vi "Remote Start.vi"(8 "error in":errorcluster, 11 "Master Controller in":refnum<class "EMS User Interface.lvclass">) -> (0 "error out":errorcluster, 3 "Master Controller out":refnum<class "EMS User Interface.lvclass">)   [LabVIEW 2018, in "EMS User Interface Actor.lvlib" / "EMS User Interface.lvclass"]
uses:
  EMS User Interface.lvclass
  EMS User Interface.lvclass/EMS User Interface.ctl
  <vilib>/ActorFramework/Message Enqueuer/Message Enqueuer.lvclass/Message Enqueuer.ctl
  <vilib>/ActorFramework/Message Enqueuer/Enqueue.vi
  EMS Core/EMS Messages/Commissioning Init Msg/Commissioning Init Msg.lvclass
  C:/Program Files (x86)/National Instruments/LabVIEW 2018/vi.lib/ActorFramework/Message/Message.lvclass
  <vilib>/ActorFramework/Message Priority Queue/Priority Enqueue.vi
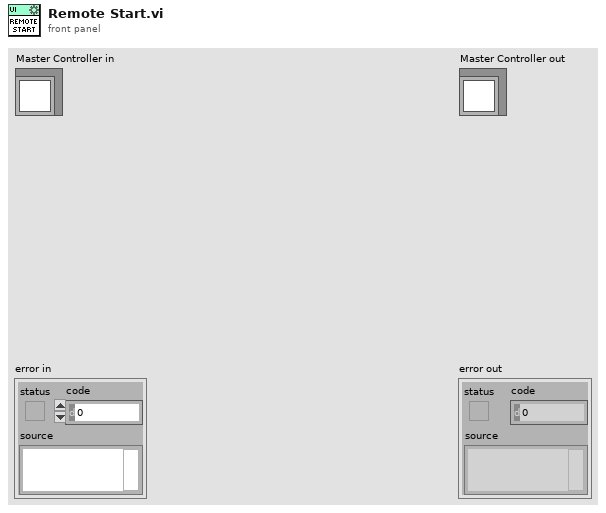
[diagram p1: front panel]
types:
  T1 = typedef "EMS Core.lvlib/EMS.lvclass/Microgrid State.ctl" = enum16{"Discovery", "Commissioning", "Activation", "Blackstart", "OnGrid", "OffGrid", "Island", "Resynchronization", "Manual", "Shutdown", "Stop"}
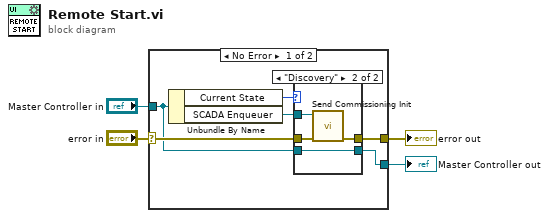
[diagram p0: block diagram]
diagram:
  n1 = case shown="No Error" "error in" {
    selector: "error in" -> [w9 w18]
    tunnel: [w10 w18] -> w2
    tunnel: [w8 w17] -> w1
    tunnel: "Master Controller in" -> [w6 w17]
    frame No Error {
      n2 = Unbundle By Name(w6) -> ("Current State"=w7:T1, "SCADA Enqueuer"=w5:refnum<class "Message Enqueuer.lvclass">)
      n3 = case shown="\"Discovery\"" w7 {
        tunnel: [w12 w14] -> w10
        tunnel: w6 -> [w11 w16]
        tunnel: w9 -> [w12 w15]
        tunnel: [w11 w16] -> w8
        tunnel: w5 -> [_ w13]
        frame "Shutdown", Default {
        }
        frame "Discovery" {
          n4 = call "Send Commissioning Init.vi"("error in (no error)"=w15, "Message Enqueuer"=w13) -> ("error out"=w14:errorcluster)  [unwired: 8 in, 1 out]
        }
      }
    }
    frame Error {
    }
  }
  "error out" <- w2
  "Master Controller out" <- w1
